vi "Get_Sub_Collection.vi"(8 "error in (no error)":errorcluster caption="entrée d'erreur (pas d'erreur)", 11 "Firebase Benches en entrée":refnum<class "Firebase AssembledProducts_Booleen.lvclass">) -> (0 "error out":errorcluster caption="sortie d'erreur", 3 "Firebase Benches en sortie":refnum<class "Firebase AssembledProducts_Booleen.lvclass">)   [LabVIEW 2020, in "Library Instrument & Equipement.lvlib" / "Library FireBase.lvlib" / "Firebase AssembledProducts_Booleen.lvclass"]
doc: "Return the documents present in the test collection for each DATA read with Get_Data\nPlease initialise the following values\n - Name BDD\n - Document of test sequence\n - API Key\n - Nb To Read"
uses:
  Firebase AssembledProducts_Booleen.lvclass
  C:/Users/ngarcin/OneDrive - Altyor/Standard TB/Class/Firebase/Source/Firebase AssembledProducts/Firebase AssembledProducts.lvclass
  C:/Users/ngarcin/OneDrive - Altyor/Standard TB/Class/Firebase/Source/Firebase Driver/Firebase Driver.lvclass
  Firebase AssembledProducts_Booleen.lvclass/Firebase AssembledProducts_Booleen.ctl
  JSON API/JSON Value/Set from JSON string.vi
  JSON API/JSON Value/JSON Value.lvclass
  Firebase AssembledProducts.lvclass
  JSON API/Variant JSON/Variant JSON.lvlib
  JSON API/Get Polymorphic/JSON GetSet.lvlib
  Firebase Driver/Firebase Driver.lvclass
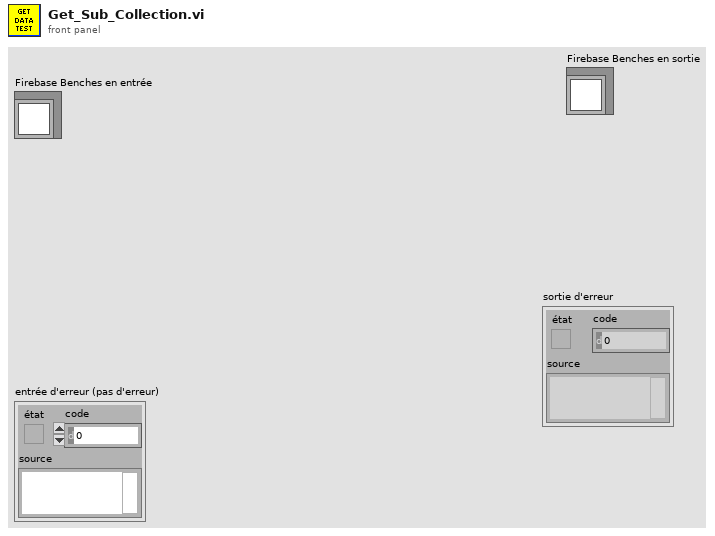
[diagram p1: front panel]
types:
  T1 = cluster{"name":string, "fields":cluster{"Result":cluster{"booleanValue":bool}, "Name":cluster{"stringValue":string}, "StartOfTest":cluster{"timestampValue":string}, "EndOfTest":cluster{"timestampValue":string}, "limit":cluster{"mapValue":cluster{"fields":cluster{"Lower":cluster{"stringValue":string}, "Upper":cluster{"stringValue":string}}}}, "Value":cluster{"booleanValue":bool}, "Type":cluster{"stringValue":string}, "MainTest":cluster{"stringValue":string}}}[][]
  T2 = cluster{"name":string, "fields":cluster{"Result":cluster{"booleanValue":bool}, "CreationDate":cluster{"timestampValue":string}, "Batch":cluster{"stringValue":string}, "SerialNumber":cluster{"stringValue":string}, "EndOfProduction":cluster{"timestampValue":string}, "FW_Version":cluster{"mapValue":cluster{"fields":cluster{"Bootloader":cluster{"mapValue":cluster{"fields":cluster{"File_Name":cluster{"stringValue":string}, "Version":cluster{"mapValue":cluster{"fields":cluster{"Major":cluster{"stringValue":string}, "Minor":cluster{"stringValue":string}}}}, "Checksum":cluster{"stringValue":string}}}}, "SoftDevice":cluster{"mapValue":cluster{"fields":cluster{"File_Name":cluster{"stringValue":string}, "Version":cluster{"mapValue":cluster{"fields":cluster{"Major":cluster{"stringValue":string}, "Minor":cluster{"stringValue":string}}}}, "Checksum":cluster{"stringValue":string}}}}, "DFU":cluster{"mapValue":cluster{"fields":cluster{"File_Name":cluster{"stringValue":string}, "Version":cluster{"mapValue":cluster{"fields":cluster{"Major":cluster{"stringValue":string}, "Minor":cluster{"stringValue":string}}}}, "Checksum":cluster{"stringValue":string}}}}}}}, "PartNumber":cluster{"stringValue":string}, "OrderNumber":cluster{"stringValue":string}, "Operator":cluster{"stringValue":string}, "AssembledProductName":cluster{"stringValue":string}}}[]
  T3 = cluster{"name":string, "fields":cluster{"Result":cluster{"booleanValue":bool}, "Name":cluster{"stringValue":string}, "StartOfTest":cluster{"timestampValue":string}, "EndOfTest":cluster{"timestampValue":string}, "limit":cluster{"mapValue":cluster{"fields":cluster{"Lower":cluster{"stringValue":string}, "Upper":cluster{"stringValue":string}}}}, "Value":cluster{"booleanValue":bool}, "Type":cluster{"stringValue":string}, "MainTest":cluster{"stringValue":string}}}[]
  T4 = cluster{"documents":cluster{"name":string, "fields":cluster{"Result":cluster{"booleanValue":bool}, "Name":cluster{"stringValue":string}, "StartOfTest":cluster{"timestampValue":string}, "EndOfTest":cluster{"timestampValue":string}, "limit":cluster{"mapValue":cluster{"fields":cluster{"Lower":cluster{"stringValue":string}, "Upper":cluster{"stringValue":string}}}}, "Value":cluster{"booleanValue":bool}, "Type":cluster{"stringValue":string}, "MainTest":cluster{"stringValue":string}}}[], "nextPageToken":string}
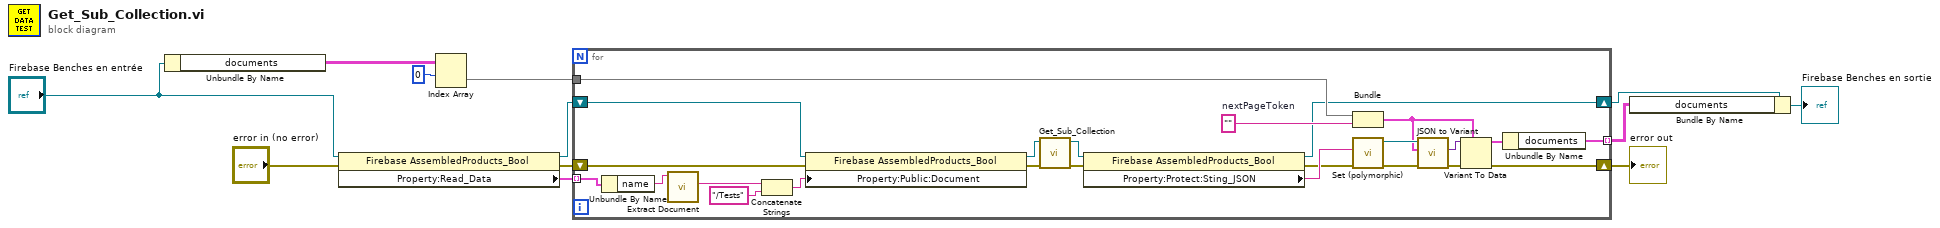
[diagram p0: block diagram]
diagram:
  n1 = Unbundle By Name("Firebase Benches en entrée") -> ("documents"=w11:T1)
  n2 = property class="Firebase AssembledProducts_Bool"(reference="Firebase Benches en entrée", error in="error in (no error)") -> (reference out=w5:refnum<class "Firebase AssembledProducts_Booleen.lvclass">, error out=w6:errorcluster, "Property:Read_Data"=w7:T2)
  n3 = Index Array(array=w11, index (row)=0 ("indice (ligne)")) -> (element=w10:T3)  [unwired: 1 in]
  n4 = for {
    tunnel: [w30] -> w12 mode=indexing
    shift-right: [w15] -> w8
    shift-left: w5 -> [w29]
    shift-right: [w18] -> w3
    shift-left: w6 -> [w28]
    tunnel: w7 -> [w27] mode=indexing
    tunnel: w10 -> [w20]
    w32 = ""  # nextPageToken
    n5 = Unbundle By Name(w27) -> ("name"=w26:string)
    n6 = call "Extract Document.vi"("Name"=w26) -> ("Source"=w25:string)  [unwired: 9 in, 1 out]
    n7 = Concatenate Strings(w25, "/Tests" ("chaîne")) -> (w23:string)
    n8 = property class="Firebase AssembledProducts_Bool"(reference=w29, error in=w28, "Property:Public:Document"=w23) -> (reference out=w21:refnum<class "Firebase AssembledProducts_Booleen.lvclass">, error out=w22:errorcluster)
    n9 = call-parent "Get_Sub_Collection.vi"("error in (no error)"=w22, "Firebase Benches en entrée"=w21) -> ("error out"=w17:errorcluster, "Firebase Benches en sortie"=w16:refnum<class "Firebase AssembledProducts_Booleen.lvclass">)  [unwired: 8 in]
    n10 = property class="Firebase AssembledProducts_Bool"(reference=w16, error in=w17) -> (reference out=w15:refnum<class "Firebase AssembledProducts_Booleen.lvclass">, error out=w13:errorcluster, "Property:Protect:Sting_JSON"=w14:string)
    n11 = Bundle("documents"=w20, "nextPageToken"=w32) -> (w31:T4)  [unwired: 1 in]
    n12 = call-poly "Set (polymorphic).vi"("error in (no error)"=w13, "JSON stream"=w14) -> ("error out"=w34:errorcluster, "JSON Value out"=w36:refnum<class "JSON Value.lvclass">)  [unwired: 7 in, 1 out]
    n13 = call "JSON to Variant.vi"("error in (no error)"=w34, "Variant (Data Type)"=w31, "JSON Value"=w36) -> ("error out"=w35:errorcluster, "Variant out"=w19:variant)  [unwired: 7 in]
    n14 = Variant To Data(error in=w35, type=w31, Variant=w19) -> (data=w33:T4, error out=w18:errorcluster)
    n15 = Unbundle By Name(w33) -> ("documents"=w30:T3)
  }
  "error out" <- w3
  n16 = Bundle By Name(cluster=w8, "documents"=w12) -> (→"Firebase Benches en sortie":refnum<class "Firebase AssembledProducts_Booleen.lvclass">)
